vi "Thor_StopImmidiate.vi"(8 "error in (no error)":errorcluster, 10 "Device In":T1, 11 "KCubeServoControl In":T2) -> (0 "error out":errorcluster, 2 "Device Out":T1, 3 "KCubeServoControl out":T2)   [LabVIEW 2020]
uses:
  Thor_KCubeServoDCRef.ctl
  E:/Norway Project/All Hardware/New Microscope/LabVIEW/ThorLabs/Thorlabs.MotionControl.Controls.dll
  Thorlabs.MotionControl.Controls.dll
  Thor_DeviceRef.ctl
  E:/Norway Project/All Hardware/New Microscope/LabVIEW/ThorLabs/ThorLabs.MotionControl.KCube.DCServoCLI.dll
  ThorLabs.MotionControl.KCube.DCServoCLI.dll
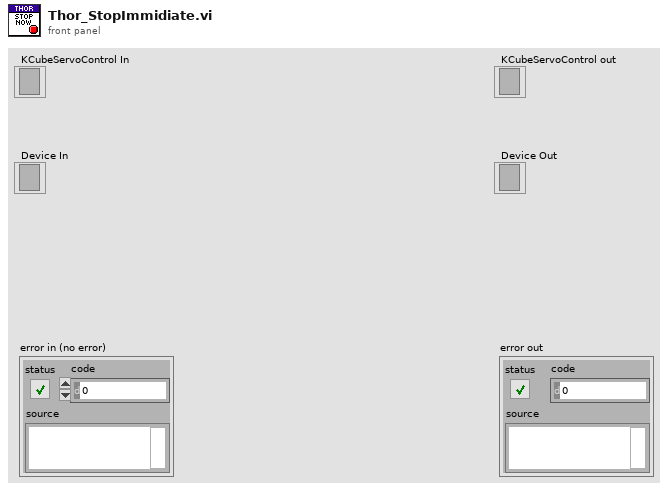
[diagram p1: front panel]
types:
  T1 = typedef "Thor_DeviceRef.ctl" = refnum<k24>
  T2 = typedef "Thor_KCubeServoDCRef.ctl" = refnum<k24>
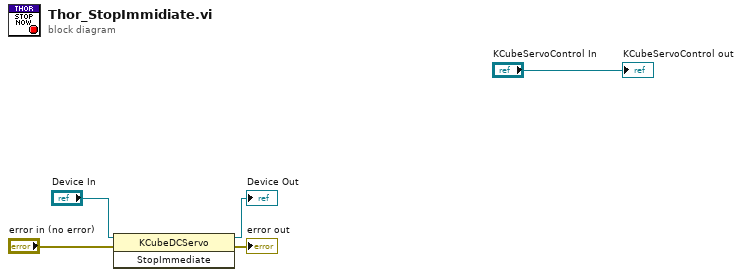
[diagram p0: block diagram]
diagram:
  n1 = invoke class="KCubeDCServo" method="StopImmediate"(reference="Device In", error in="error in (no error)") -> (reference out=→"Device Out":T1, error out=→"error out":errorcluster)  [unwired: 1 in, 1 out]
  "KCubeServoControl out" <- "KCubeServoControl In"
